vi "To And From String Array Test.vi"() -> (0 "error out":errorcluster, 3 "Pass":bool)   [LabVIEW 2015, in "Numeric Limit Compare Tests.lvlib"]
uses:
  Numeric Limit Compare Tests.lvlib
  Config/Numeric Limit Compare Config.lvclass
  <vilib>/NI/Tag Bus/tag/Data Type.ctl
  <vilib>/NI/Tag Bus Module Framework/channel/channel classification.ctl
  Config/Comparison Types.ctl
  Config/Numeric Limit Compare Config.lvclass/Numeric Limit Compare Config.ctl
  Config/Write channel.vi
  Config/Write Comparison Type.vi
  Config/Write Upper Limit_Limit.vi
  Config/Write Lower Limit.vi
  Config/Write Negate Result.vi
  Config/Write Result Channel.vi
  <vilib>/NI/Tag Bus/tag/tag descriptor.lvclass
  <vilib>/NI/Tag Bus Module Framework/channel/TBM channel.lvclass
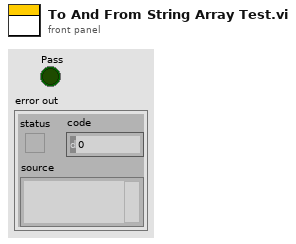
[diagram p1: front panel]
types:
  T1 = typedef "TBM channel.lvclass/channel classification.ctl" = enum16{"input data", "output data", "processing parameter", "processing result"}
  T2 = typedef "tag bus.lvlib/tag descriptor.lvclass/Data Type.ctl" = enum16{"Double", "Single", "I64", "I32", "I16", "I8", "U64", "U32", "U16", "U8", "Boolean", "String", "Array of Double", "Array of Single", "Array of I64", "Array of I32", "Array of I16", "Array of I8", "Array of U64", "Array of U32", "Array of U16", "Array of U8", "Array of Boolean", "Array of String"}
  T3 = typedef "Comparison Types.ctl" = enum16{"GELE (>=<=)", "GTLE(><=)", "GTLT(><)", "GELT(>=<)", "EQ(==)", "NE (!=)", "GT(>)", "LT(<)", "GE(>=)", "LE(<=)"}
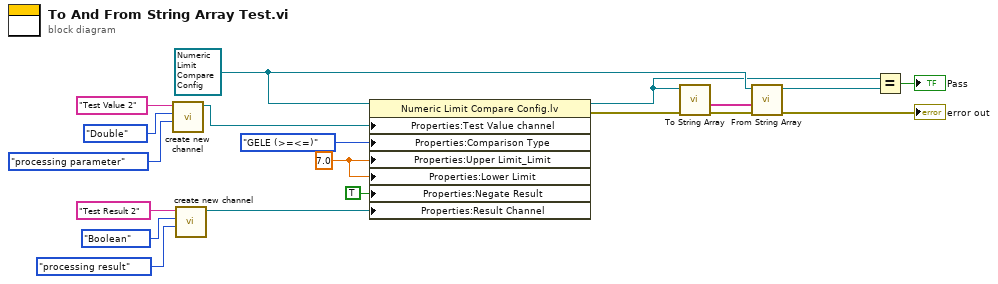
[diagram p0: block diagram]
diagram:
  w10 = 7.0 ("Upper Limit_Limit")
  w7 = refnum<class "Numeric Limit Compare Config.lvclass"> refnum ("Numeric Limit Compare Config.lvclass")
  n1 = call <vilib>:"create new channel.vi"("channel classification"=channel_classification."processing parameter", "data type"=Data_Type."Double" ("Data Type"), "channel name"="Test Value 2" ("Jump Tag Name")) -> ("channel"=w12:refnum<class "TBM channel.lvclass">)  [unwired: 8 in]
  n2 = call <vilib>:"create new channel.vi"("channel classification"=channel_classification."processing result", "data type"=Data_Type."Boolean" ("Data Type"), "channel name"="Test Result 2" ("Jump Tag Name")) -> ("channel"=w1:refnum<class "TBM channel.lvclass">)  [unwired: 8 in]
  n3 = property class="Numeric Limit Compare Config.lv"(reference=w7, "Properties:Test Value channel"=w12, "Properties:Comparison Type"=Comparison_Types."GELE (>=<=)" ("Comparison Type"), "Properties:Upper Limit_Limit"=w10, "Properties:Lower Limit"=w10, "Properties:Negate Result"=TRUE ("Negate Result"), "Properties:Result Channel"=w1) -> (reference out=w6:refnum<class "Numeric Limit Compare Config.lvclass">, error out=w18:errorcluster)  [unwired: 1 in]
  n4 = call-dynamic "To String Array.vi"("error in (no error)"=w18, "Numeric Limit Compare Config in"=w6) -> ("error out"=w19:errorcluster, "Step String Array"=w17:string[])  [unwired: 7 in, 1 out]
  n5 = call-dynamic "From String Array.vi"("error in (no error)"=w19, "String Array"=w17, "Numeric Limit Compare Config in"=w7) -> ("error out"=→"error out":errorcluster, "Numeric Limit Compare Config out"=w5:refnum<class "Numeric Limit Compare Config.lvclass">)  [unwired: 5 in, 2 out]
  n6 = Equal?(x=w6, y=w5) -> (x = y?=→"Pass":bool)
